vi "OP300ZP_SCANequipements.vi"(8 "Errin":errorcluster caption="errin", 10 "Chaîne":string="Log et conf\\Config.ini", 11 "pathin":path=path "D:/CODE/02 SLIM ZEN") -> (0 "error out":errorcluster, 1 "KO?":bool=TRUE, 2 "BT3562":refnum<visa-resource-name>, 4 "ISO OCV":string, 5 "MX5060":refnum<visa-resource-name>, 6 "ISO SPI":string="COM8", 7 "ST5520":refnum<visa-resource-name>)   [LabVIEW 2020]
doc: "Ce vi il détecte la presence des équipements"
uses:
  OP500/VG/VG_ST5520.vi
  VG/VG_BT3562.vi
  VG/VG_ARDUINO.vi
  VG/VG_MX5060.vi
  VG/ISOOCV.vi
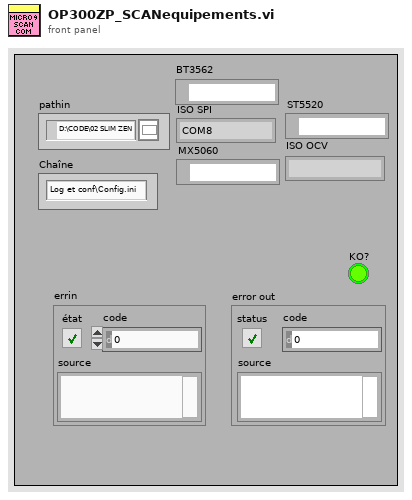
[diagram p1: front panel]
types:
  T1 = cluster{"3562":string, "MX5060":string, "ST5520":string, "ARDUINO":string}
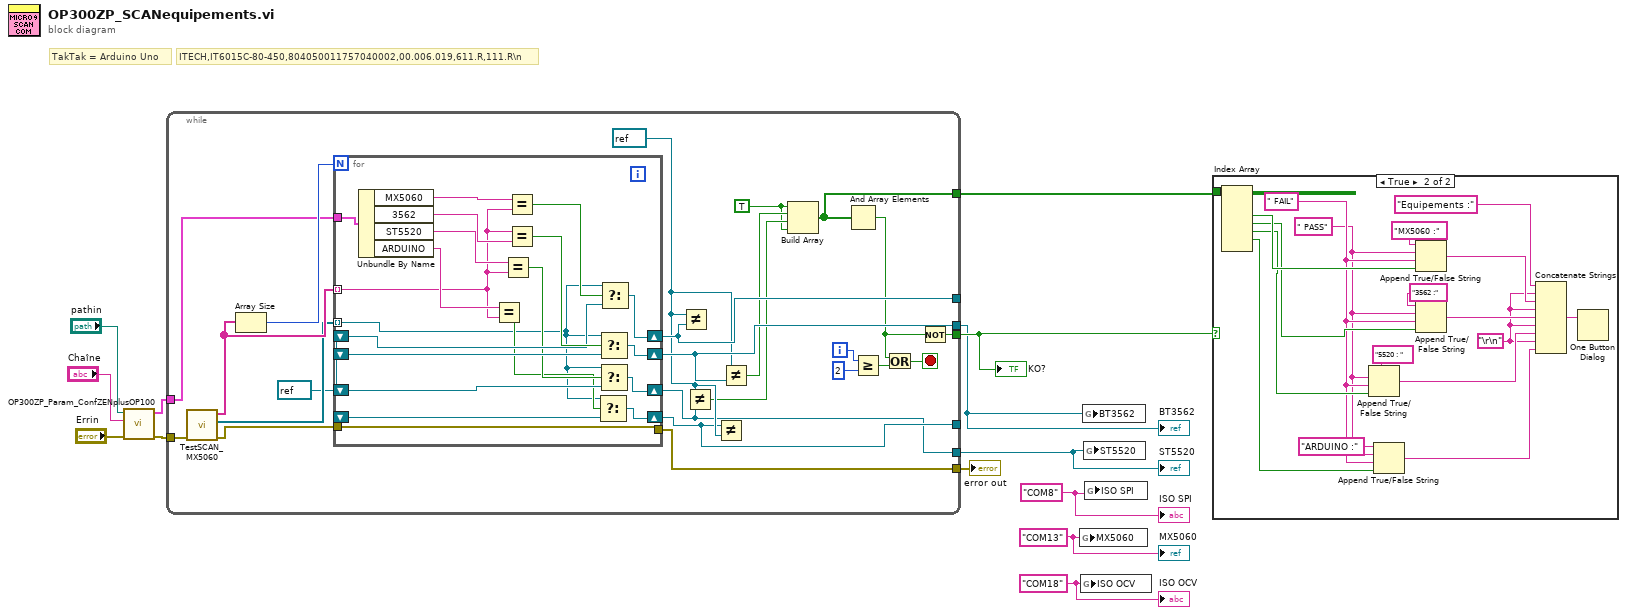
[diagram p0: block diagram]
diagram:
  w4 = "COM18" ("ISO OCV")
  w6 = "COM13" ("ARDUINO")
  w5 = "COM8" ("ARDUINO")
  # "TakTak = Arduino Uno"
  # "ITECH,IT6015C-80-450,804050011757040002,00.006.019,611.R,111.R\\n"
  n1 = call "OP300ZP_Param_ConfZENplusOP100.vi"("errin"="Errin", "Chaîne"="Chaîne", "pathin"="pathin") -> ("errout"=w10:errorcluster, "VISA OUT"=w9:T1)  [unwired: 7 in]
  n2 = while {
    tunnel: [w26] -> _
    tunnel: [w25] -> w2
    tunnel: w10 -> [w35]
    tunnel: [w30] -> w13
    tunnel: w9 -> [w27]
    tunnel: [w23] -> w12
    tunnel: [w17] -> w3
    tunnel: [w20] -> w1
    tunnel: [w18] -> _
    i -> [w29]
    stop <- w32 stop-if-true
    w14 = TRUE ("élément")
    w19 = refnum<visa-resource-name> refnum ("x")
    w22 = refnum<visa-resource-name> refnum ("VISA resource name out")
    n3 = call "TestSCAN_MX5060.vi"("errin"=w35) -> ("error out"=w21:errorcluster, "Tableau 2"=w33:refnum<visa-resource-name>[], "Tableau"=w34:string[])  [unwired: 8 in]
    n4 = Array Size(array=w34) -> (size(s)=w36:i32)
    n5 = for {
      N: w36 -> [_]
      shift-right: [w54] -> w26
      shift-left: w22 -> [w52]
      shift-right: [w53] -> w25
      shift-left: w22 -> [w51]
      tunnel: w34 -> [w41] mode=indexing
      tunnel: w27 -> [w50]
      shift-right: [w47] -> w17
      shift-left: w22 -> [w48]
      tunnel: w33 -> [w39] mode=indexing
      tunnel: w21 -> [w43]
      tunnel: [w43] -> w20
      shift-right: [w37] -> w18
      shift-left: _ -> [w38]
      n6 = Unbundle By Name(w50) -> ("MX5060"=w49:string, "3562"=w44:string, "ST5520"=w46:string, "ARDUINO"=w42:string)
      n7 = Equal?(x=w42, y=w41) -> (x = y?=w40:bool)
      n8 = Equal?(x=w46, y=w41) -> (x = y?=w45:bool)
      n9 = Equal?(x=w49, y=w41) -> (x = y?=w55:bool)
      n10 = Equal?(x=w41, y=w44) -> (x = y?=w56:bool)
      n11 = Select(t=w39, s=w40, f=w38) -> (s? t:f=w37:refnum<visa-resource-name>)
      n12 = Select(t=w39, s=w56, f=w51) -> (s? t:f=w53:refnum<visa-resource-name>)
      n13 = Select(t=w39, s=w45, f=w48) -> (s? t:f=w47:refnum<visa-resource-name>)
      n14 = Select(t=w39, s=w55, f=w52) -> (s? t:f=w54:refnum<visa-resource-name>)
    }
    n15 = Not Equal?(x=w19, y=w26) -> ()  [unwired: 1 out]
    n16 = Not Equal?(x=w19, y=w17) -> (x != y?=w15:bool)
    n17 = Not Equal?(x=w18, y=w19) -> ()  [unwired: 1 out]
    n18 = Not Equal?(x=w19, y=w25) -> (x != y?=w16:bool)
    n19 = Build Array(w14, w16, w15, w14) -> (w23:bool[])
    n20 = And Array Elements(Boolean array=w23) -> (logical AND=w24:bool)
    n21 = Greater Or Equal?(x=w29, y=2) -> (x >= y?=w31:bool)
    n22 = Or(x=w24, y=w31) -> (x .or. y?=w32:bool)
    n23 = Not(x=w24) -> (.not. x?=w30:bool)
  }
  "KO?" <- w13
  "BT3562" <- w2
  "ST5520" <- w3
  "error out" <- w1
  n24 = global write "VG_MX5060.vi" "MX5060"(w6) -> ()
  n25 = global write "ISOOCV.vi" "ISO OCV"(w4) -> ()
  n26 = global write "VG_BT3562.vi" "BT3562"(w2) -> ()
  n27 = global write "VG_ST5520.vi" "ST5520"(w3) -> ()
  n28 = global write "VG_ARDUINO.vi" "ISO SPI"(w5) -> ()
  n29 = case shown="True" w13 {
    tunnel: w12 -> [_ w66]
    frame False {
    }
    frame True {
      w58 = "\r\n"
      w60 = " PASS" ("chaîne faux")
      w61 = " FAIL" ("chaîne faux")
      n30 = Index Array(array=w66) -> (element #2=w65:bool, element #3=w64:bool, element #4=w63:bool, element #5=w62:bool)  [unwired: 6 in, 2 out]
      n31 = Append True/False String(1:w63, 2:w61, 3:w60, 4:"5520 : " ("chaîne (\"\")")) -> (0:w68:string)
      n32 = Append True/False String(1:w62, 2:w61, 3:w60, 4:"ARDUINO :" ("chaîne (\"\")")) -> (0:w57:string)
      n33 = Append True/False String(1:w65, 2:w61, 3:w60, 4:"MX5060 :" ("chaîne (\"\")")) -> (0:w70:string)
      n34 = Append True/False String(1:w64, 2:w61, 3:w60, 4:"3562 :" ("chaîne (\"\")")) -> (0:w69:string)
      n35 = Concatenate Strings("Equipements :" ("chaîne"), w58, w70, w58, w69, w58, w68, w58, w57) -> (w67:string)
      n36 = One Button Dialog(message=w67) -> ()  [unwired: 1 in, 1 out]
    }
  }
  "MX5060" <- w6
  "ISO SPI" <- w5
  "ISO OCV" <- w4
